vi "Append Table Contents to Word Bookmark.vi"(6 "mode (entire row)":enum16{"entire row", "entire column"}(ring), 7 "bookmark (word)":string, 8 "error in (no error)":errorcluster, 10 "table row contents":string[][](array[string]), 11 "report in":refnum<class "NI_report.lvclass">) -> (0 "error out":errorcluster, 3 "report out":refnum<class "NI_report.lvclass">)   [LabVIEW 2018, in "WordReportGeneration.lvlib" / "Word_Report.lvclass"]
uses:
  Word_Report.lvclass
  <vilib>/Utility/NIReport.llb/NI_report.lvclass
  <vilib>/Utility/NIReport.llb/Word/NI_Word.lvclass
  WordReportGeneration.lvlib
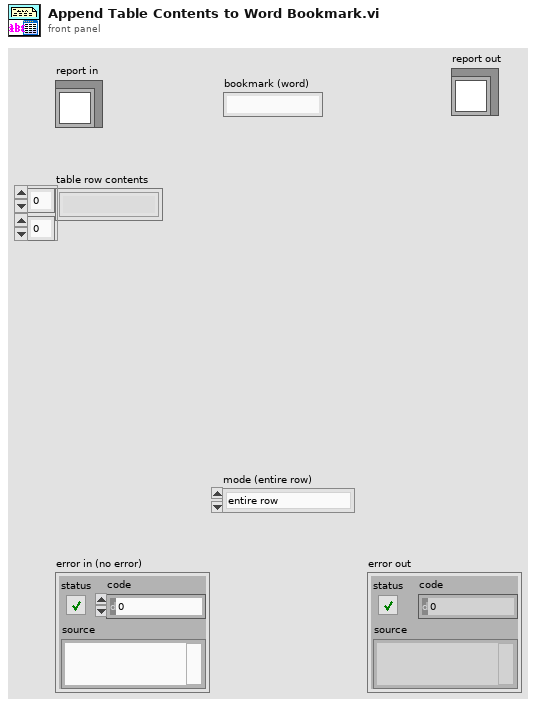
[diagram p1: front panel]
types:
  T1 = cluster{"position (Excel)":cluster{"row":i32, "column":i32}, "name (Excel) ":string, "bookmark (Word)":string}
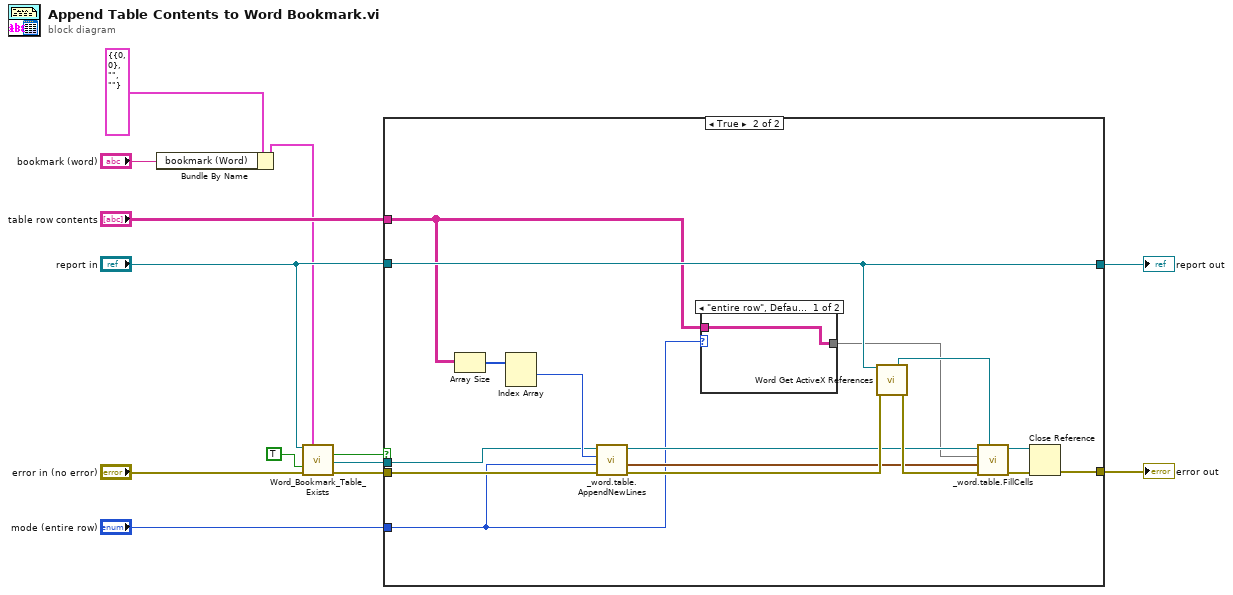
[diagram p0: block diagram]
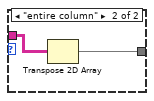
[diagram p3: hidden frame]
diagram:
  n1 = Bundle By Name(cluster=T1 {"position (Excel)"={"row"=0, "column"=0}, "name (Excel) "="", "bookmark (Word)"=""} ("MS Office parameters"), "bookmark (Word)"="bookmark (word)") -> (w5:T1)
  n2 = call <vilib>:"Word_Bookmark_Table_Exists.vi"("report in"="report in", "MS Office parameters"=w5, "get table ref?"=TRUE, "error in (no error)"="error in (no error)") -> ("bookmark to existing table?"=w3:bool, "table ref"=w8:refnum<k7>, "error out"=w9:errorcluster)  [unwired: 8 in, 1 out]
  n3 = case shown="True" w3 {
    tunnel: "report in" -> [w14 w22]
    tunnel: [w15 w31] -> w12
    tunnel: "table row contents" -> [_ w16]
    tunnel: w8 -> [_ w27]
    tunnel: "mode (entire row)" -> [_ w18]
    tunnel: w9 -> [w15 w28]
    tunnel: [w14 w22] -> w1
    frame False {
    }
    frame True {
      n4 = Array Size(array=w16) -> (size(s)=w29:i32[])
      n5 = Index Array(array=w29) -> (element #1=w30:i32)  [unwired: 2 in, 1 out]
      n6 = call "_word.table.AppendNewLines.vi"("error in (no error)"=w28, "mode"=w18, "number"=w30, "table Refnum in"=w27) -> ("error out"=w23:errorcluster, "Cluster"=w19:cluster{"x+1":i32, "x+1":i32}, "table Refnum out"=w21:refnum<k7>)  [unwired: 5 in]
      n7 = case shown="\"entire row\", Default" w18 {
        tunnel: w16 -> [w32 w34]
        tunnel: [w32 w33] -> w17
        frame "entire row", Default {
        }
        frame "entire column" {
          n8 = Transpose 2D Array(2D array=w34) -> (transposed array=w33:string[][])
        }
      }
      n9 = call <vilib>:"Word Get ActiveX References.vi"("report in"=w22, "error in (no error)"=w23) -> ("Word._Application"=w20:refnum<k7>, "error out"=w24:errorcluster)  [unwired: 7 in, 5 out]
      n10 = call "_word.table.FillCells.vi"("word.application"=w20, "error in (no error)"=w24, "start cell"=w19, "table row contents"=w17, "table in"=w21) -> ("error out"=w25:errorcluster, "table out"=w26:refnum<k7>)  [unwired: 5 in]
      n11 = Close Reference(reference=w26, error in (no error)=w25) -> (error out=w31:errorcluster)
    }
  }
  "error out" <- w12
  "report out" <- w1
